vi "ConvertPercentToPressure.vi"(10 "Measure Percentage":dbl, 11 "Full Scale (bar a)":dbl) -> (3 "Pressure (bar a)":dbl)   [LabVIEW 2019]
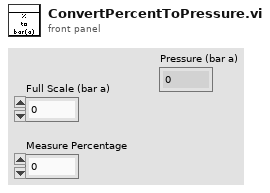
[diagram p1: front panel]
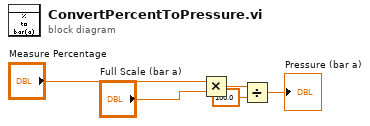
[diagram p0: block diagram]
diagram:
  n1 = Multiply(x="Measure Percentage", y="Full Scale (bar a)") -> (x*y=w4:dbl)
  n2 = Divide(x=w4, y=100.0) -> (x/y=→"Pressure (bar a)":dbl)
